vi "DB - [MasterData].[Procedure].vi"(0 "connection reference":T5, 1 "DB Connection":T1={"Open"=TRUE, "Close"=TRUE}, 2 "DB - Master Data Enum":T2, 5 "DB.Schema.Table\nSRTRS.MasterData.Procedure":string="SRTRS.MasterData.Procedure", 7 "Include Inactive":bool=TRUE, 9 "DB.Schema.Table\nSRTRS.MasterData.ProcedureItem":string="SRTRS.MasterData.ProcedureItem", 11 "error in (no error)":errorcluster, 12 "MCListbox Refnum":refnum<vi>, 13 "Clust Refnum":refnum<vi>, 14 "CmbBox Refnum":refnum<vi>) -> (4 "connection reference":T5, 6 "Result":string[](array[string]), 8 "ItemNames":string[][](array[string]), 15 "SUMMARY":errorcluster)   [LabVIEW 2013]
uses:
  <vilib>/addons/database/Connection.llb/Conn ObjectReference.ctl
  Controls/Combo Box.ctl
  Controls/DB - Master Data Procedure Enum.ctl
  Controls/DB - OpenClose.ctl
  Controls/Global SRTRS.vi
  <vilib>/addons/database/Connection.llb/DB Tools Open Connec (String).vi
  <vilib>/addons/database/Connection.llb/Conn Execute.vi
  <vilib>/addons/database/Recordset.llb/Rec Destroy - Connection.vi
  <vilib>/addons/database/Recordset.llb/Rec Fetch Recordset Data (R).vi
  <vilib>/addons/database/_DB Variant To Data/Database Variant To Data.xnode
  <vilib>/addons/database/NI_Database_API.lvlib
panel:
  out "Refnum":errorcluster
  out "Close":errorcluster
  out "Not a Refnum?":bool
  out "array w/ subset deleted":string[][](array[string])
  out "revision":string[][](array[string])
  in  "MCListBox FHS Master Data":i32(listbox)=-1 caption="Furnance Heating Sequence"
  out "SQL Statement":errorcluster
  out "ms":u32=3
  out "SQL Statement":string="USE [SRTRS]\n--GO\n\nINSERT INTO [MasterData].[Procedure]\n           ([procedureNo]\n           ,[revision]\n           ,[holdTemperture]\n           ,[unitOfMeasurement]\n           ,[holdTimeDuration]\n           ,[def]\n           ,[createdBy]\n           ,[createdOn]\n           ,[lastSavedBy]\n           ,[lastSavedOn]\n           ,[Inactive])\n     VALUES\n           ('WPS5' ,'2' ,'32' ,'°C' ,'00:02' ,'' ,'User' ,'2014-08-29 16:57:39' ,'User' ,'2014-08-29 16:57:39' ,'0' )\n--GO\n"
  in  "WPS Details Master Data":T4={"Master Data WPS/Ref"="WPS5", "Master Data Rev"="2", "Master Data Hold Temperature"="32", "Master Data Temperature Units"="°C", "Master Data Hold Time (HH:MM)"="00:02", "Inactive"=FALSE} caption="Header"
  out "procedureNo":string[][](array[string])=[["2", "1", "1", "20", "", "2014-08-29 14:24:57", "", "", "", "", "", ""]]
  out "Connection Information":T6={"Connection "="SQL Server 32bit HPEnvy", "Username"="admin", "Password"="admin123"}
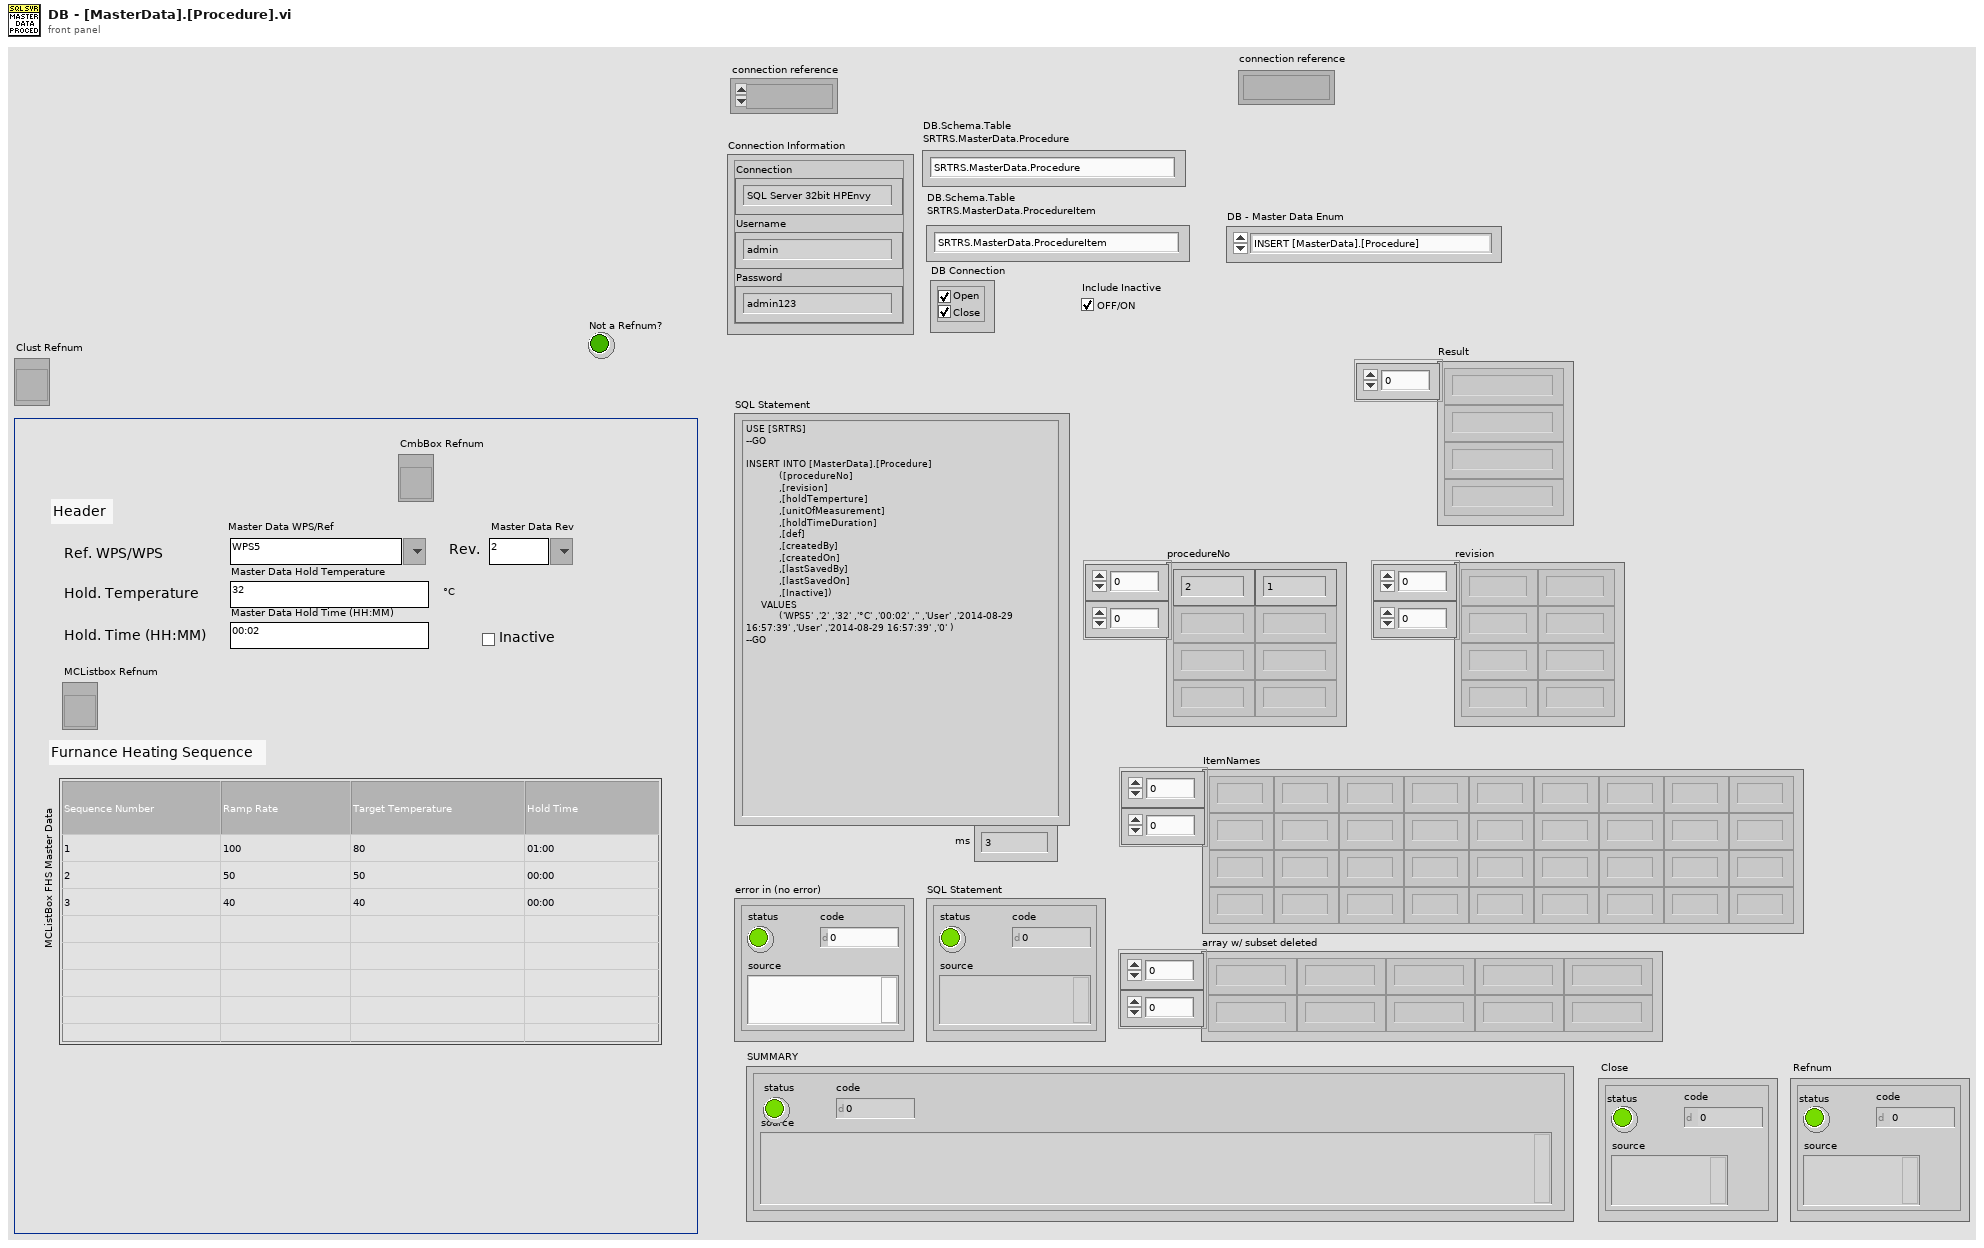
[diagram p1: front panel]
types:
  T1 = typedef "DB - OpenClose.ctl" = cluster{"Open":bool, "Close":bool}
  T2 = typedef "DB - Master Data Procedure Enum.ctl" = enum16{"INSERT [MasterData].[Procedure]", "INSERT [MasterData][ProcedureItem]", "SELECT [ProcedureNo]", "SELECT [ProcedureRev]", "SELECT [MasterData].[ProcedureItem]"}
  T3 = typedef "Combo Box.ctl" = string
  T4 = cluster{"Master Data WPS/Ref":T3, "Master Data Rev":T3, "Master Data Hold Temperature":string, "Master Data Temperature Units":string, "Master Data Hold Time (HH:MM)":string, "Inactive":bool}
  T5 = typedef "NI_Database_API.lvlib/Conn ObjectReference.ctl" = refnum<k1>
  T6 = cluster{"Connection ":string, "Username":string, "Password":string}
  T7 = typedef "Enum - InteractiveMode-SubVIMode.ctl" = enum16{"Interactive", "subVI Mode"}
  T8 = typedef "DB - Logon Info.ctl" = cluster{"PlantID":string, "SystemID":string, "UserID":string, "DomainID":string, "LanguageID":string, "StationID":string}
  T9 = typedef "Connection Information Cluster.ctl" = cluster{"Connection ":string, "Username":string, "Password":string}
  T10 = typedef "DB - DB.Schema.Table.ctl" = cluster{"DB":string, "Schema":string, "Table":string}
  T11 = typedef "NI_Database_API.lvlib/Rec ObjectReference.ctl" = refnum<k1>
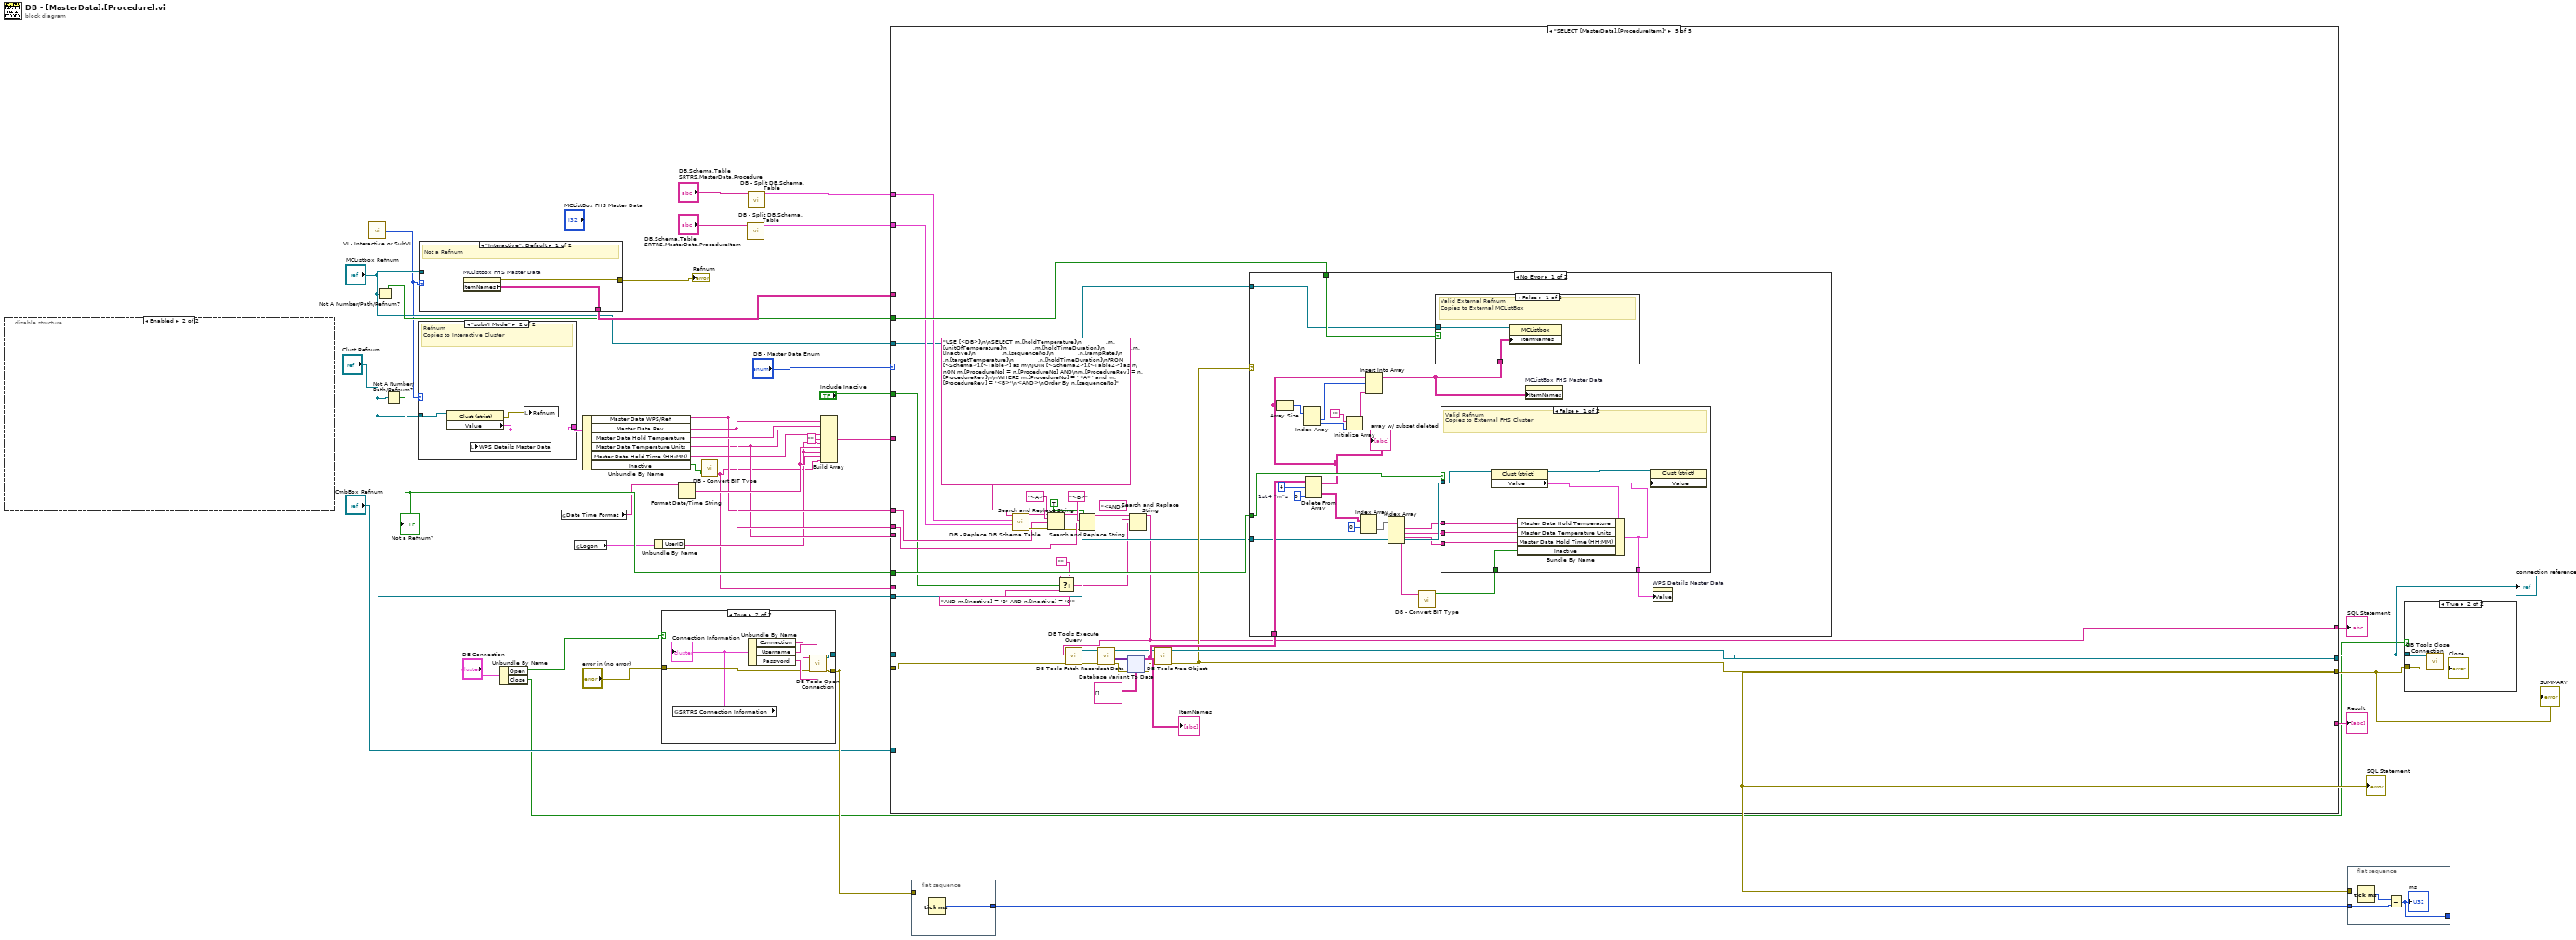
[diagram p0: block diagram]
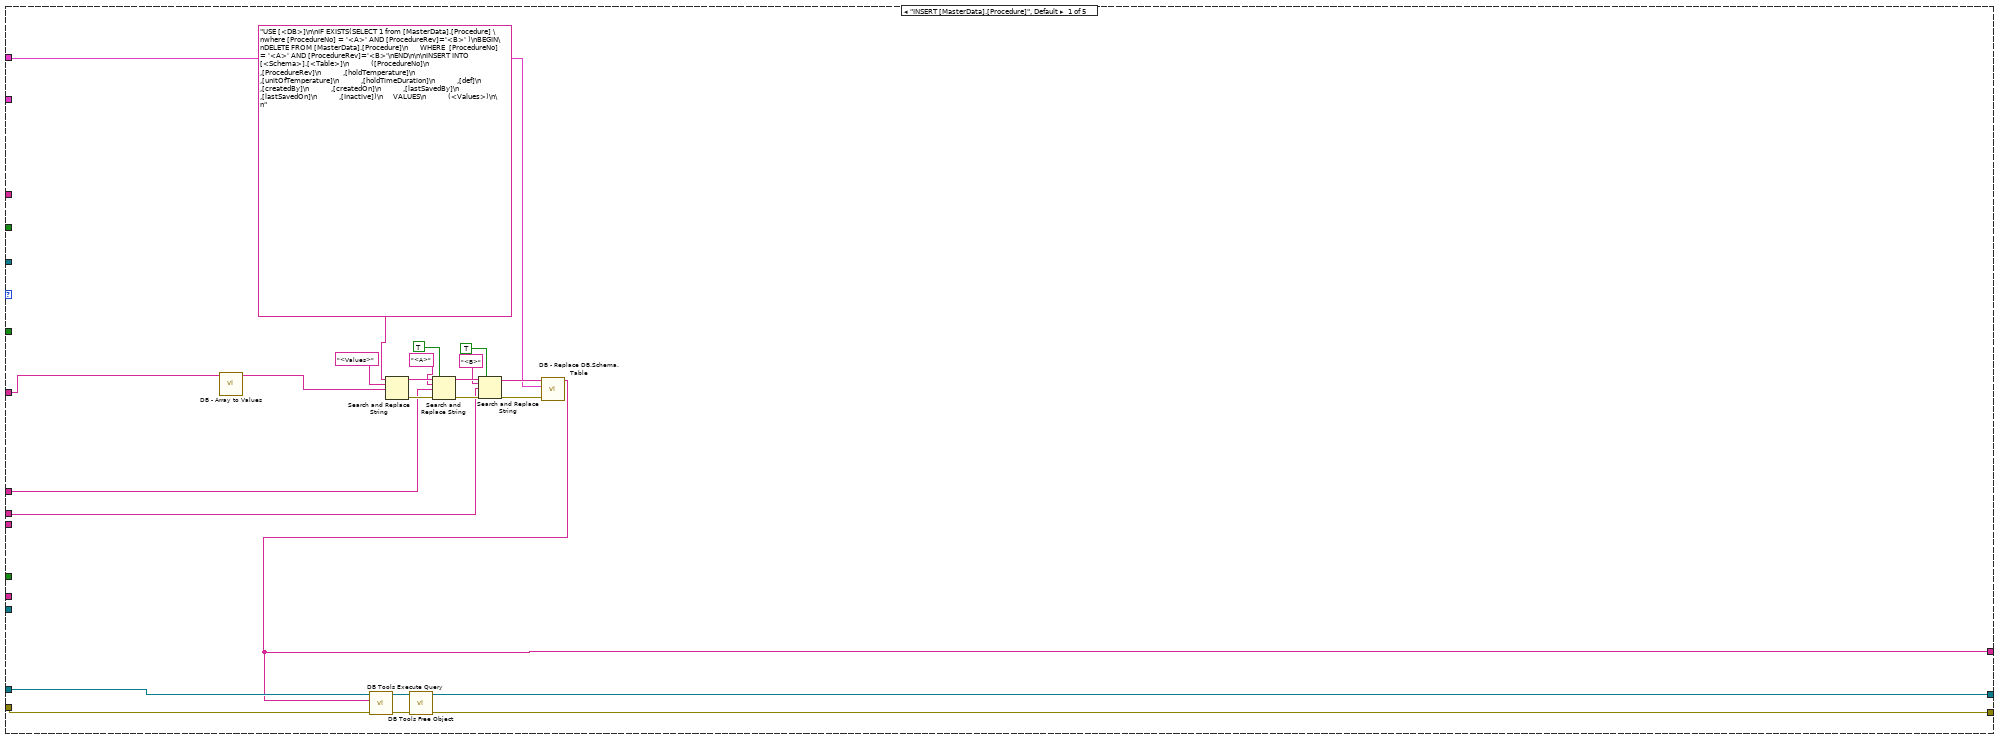
[diagram p3: hidden frame]
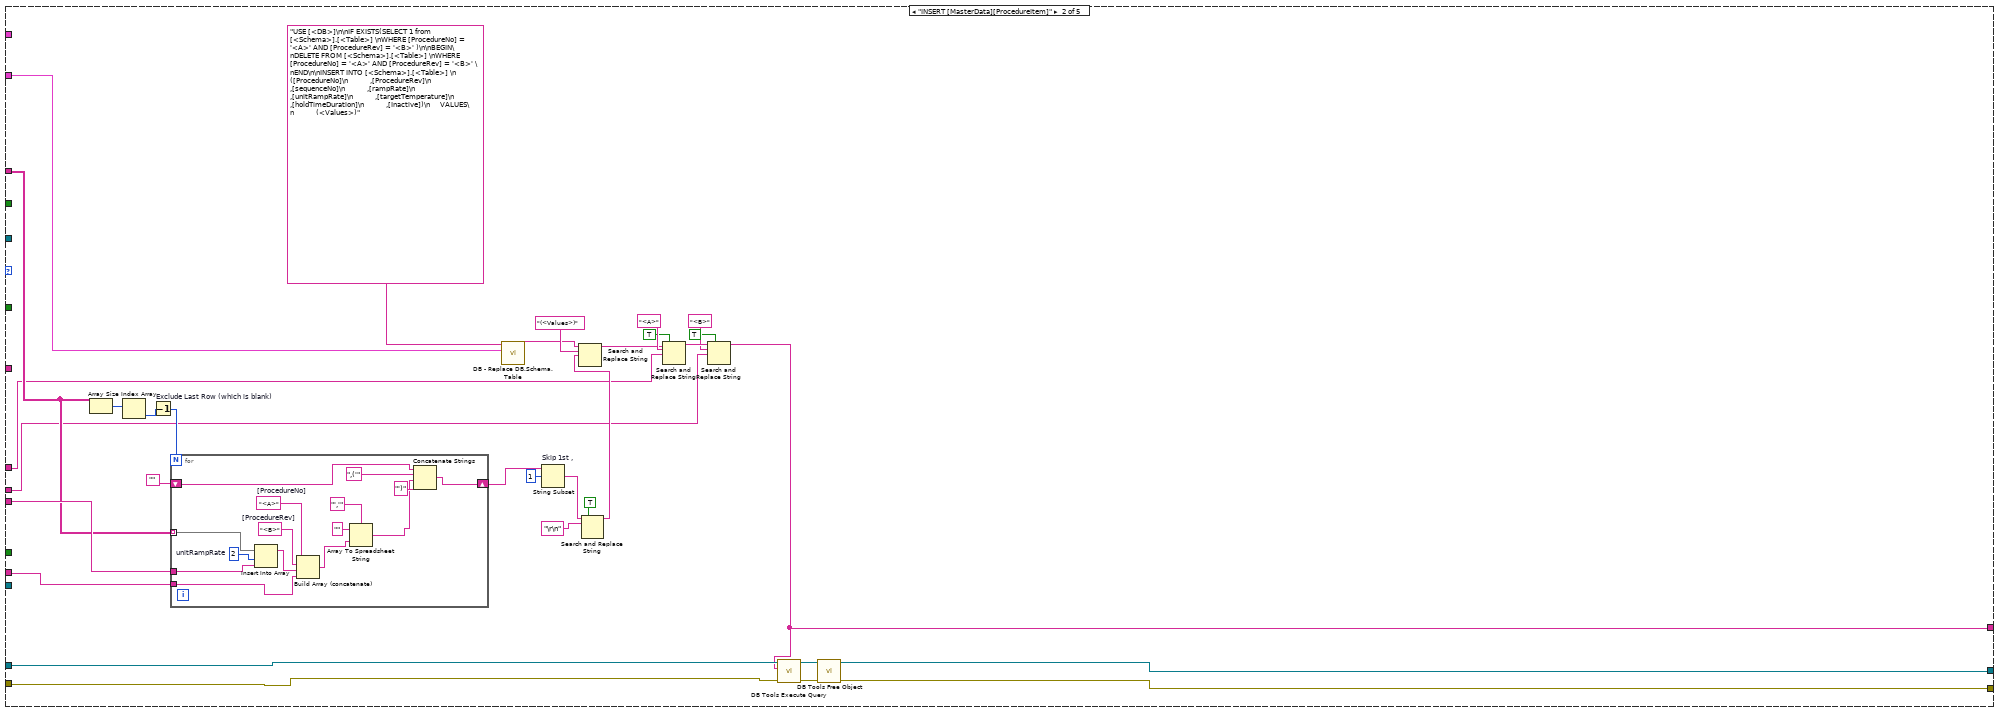
[diagram p4: hidden frame]
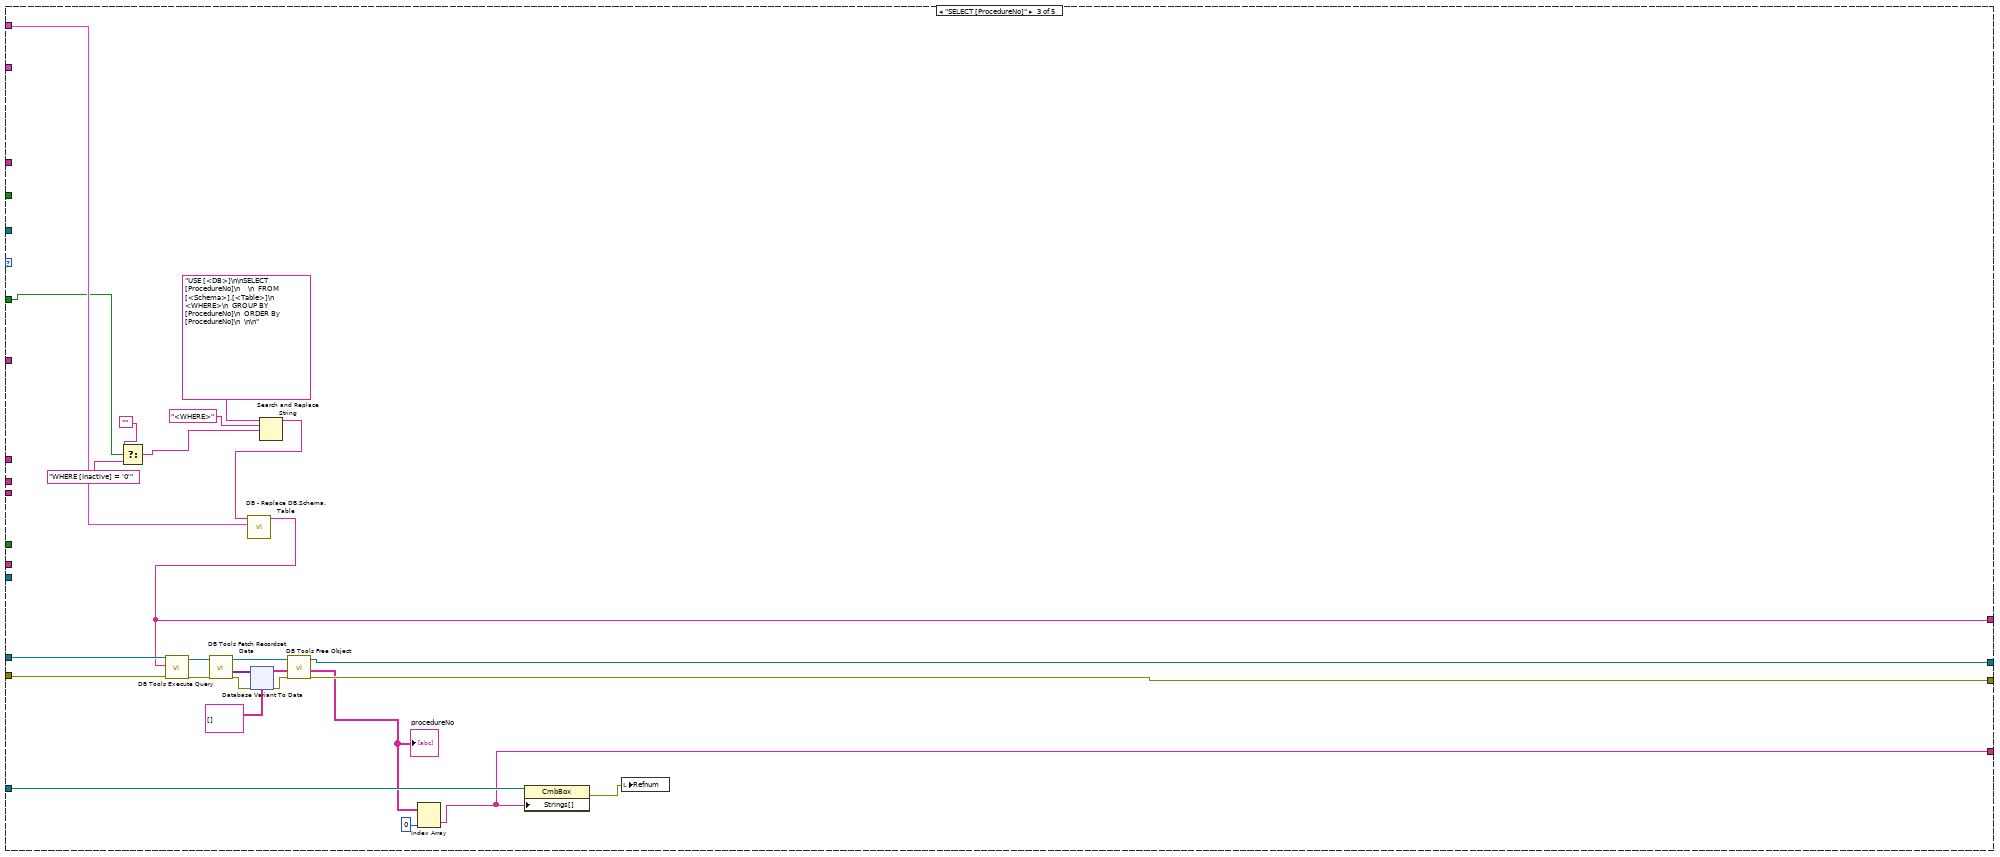
[diagram p5: hidden frame]
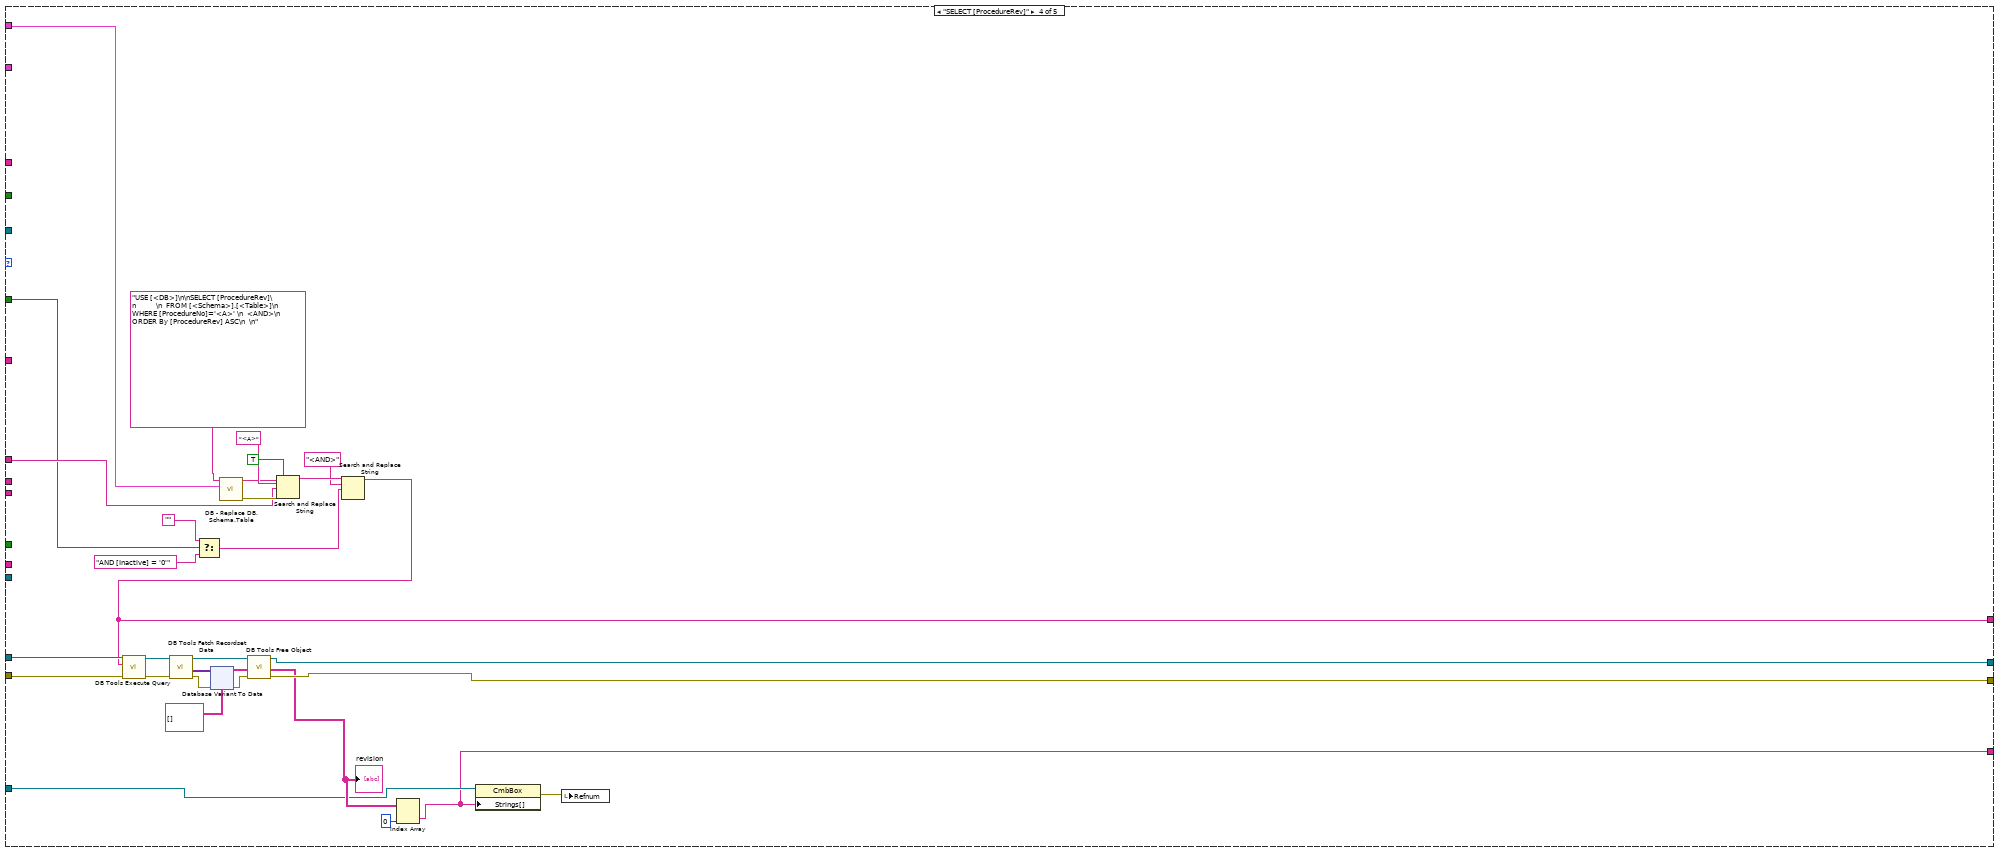
[diagram p6: hidden frame]
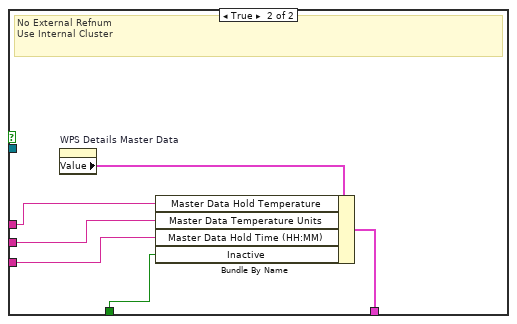
[diagram p7: hidden frame]
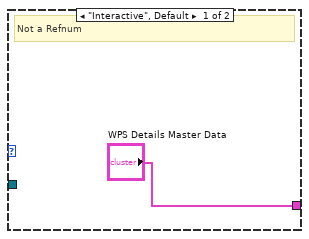
[diagram p10: hidden frame]
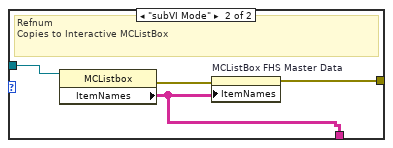
[diagram p11: hidden frame]
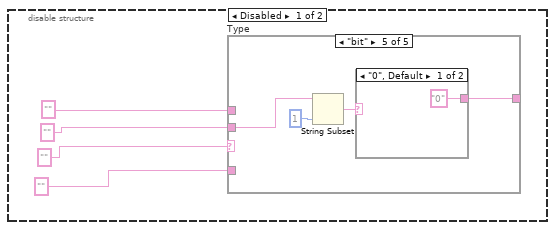
[diagram p12: hidden frame]
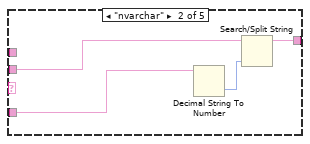
[diagram p14: hidden frame]
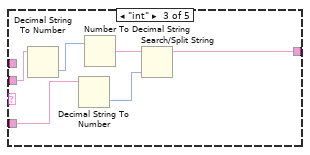
[diagram p15: hidden frame]
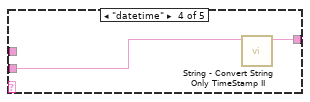
[diagram p16: hidden frame]
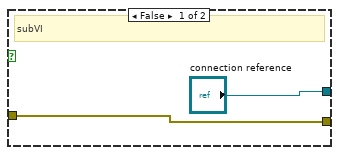
[diagram p18: hidden frame]
diagram:
  n1 = disable-structure shown="Enabled" {
    frame Disabled {
      n2 = case "Type" shown="\"bit\"" "" {
        tunnel: "" -> [w44 w47 w54 w56 w60]
        tunnel: "" -> [_ _ _ _ _]
        tunnel: "" -> [_ w46 w50 _ _]
        tunnel: [w44 w45 w49 w55 w57] -> _
        frame "False", Default {
        }
        frame "nvarchar" {
          n3 = Decimal String To Number(string=w46) -> (number=w48:i32)  [unwired: 2 in, 1 out]
          n4 = Search/Split String(string=w47, offset (0)=w48) -> (substring before match=w45:string)  [unwired: 1 in, 2 out]
        }
        frame "int" {
          n5 = Decimal String To Number(string=w54) -> (number=w53:i32)  [unwired: 2 in, 1 out]
          n6 = Decimal String To Number(string=w50) -> (number=w52:i32)  [unwired: 2 in, 1 out]
          n7 = Number To Decimal String(number=w53) -> (decimal integer string=w51:string)  [unwired: 1 in]
          n8 = Search/Split String(string=w51, offset (0)=w52) -> (substring before match=w49:string)  [unwired: 1 in, 2 out]
        }
        frame "datetime" {
          n9 = call "String - Convert String Only TimeStamp II.vi"("YYYY-mm-dd HH:MM:SS"=w56) -> ("YYYY-mm-dd HH:MM:SS"=w55:string)  [unwired: 9 in, 1 out]
        }
        frame "bit" {
          n10 = String Subset(string=w60, length (rest)=1 ("length (rest)")) -> (substring=w58:string)  [unwired: 1 in]
          n11 = case shown="\"0\", Default" w58 {
            selector: w58 -> [_ w62]
            tunnel: ["0" w62] -> w57
            frame "0", Default {
            }
            frame "1" {
            }
          }
        }
      }
    }
    frame Enabled {
    }
  }
  n12 = call "VI - Interactive or SubVI.vi"() -> ("Mode"=w9:T7)  [unwired: 5 in]
  n13 = Not A Number/Path/Refnum?(number/path/refnum="MCListbox Refnum") -> (NaN/Path/Refnum?=w19:bool)
  n14 = Not A Number/Path/Refnum?(number/path/refnum="Clust Refnum") -> (NaN/Path/Refnum?=w14:bool)
  "Not a Refnum?" <- w14
  n15 = case shown="\"subVI Mode\"" w9 {
    tunnel: "Clust Refnum" -> [_ w66]
    tunnel: ["WPS Details Master Data" w65] -> w27
    frame "Interactive", Default {
      # "Not a Refnum"
    }
    frame "subVI Mode" {
      # "Refnum\nCopies to Interactive Cluster"
      n16 = property class="Clust (strict)"(reference=w66) -> (error out=w64:errorcluster, "Value"=w65:T4)  [unwired: 1 in, 1 out]
      n17 = local write "WPS Details Master Data"(w65) -> ()
      n18 = local write "Refnum"(w64) -> ()
    }
  }
  n19 = case shown="\"Interactive\", Default" w9 {
    tunnel: "MCListbox Refnum" -> [_ w72]
    tunnel: [w68 w71] -> w22
    tunnel: [w67 w69] -> w8
    frame "Interactive", Default {
      # "Not a Refnum"
      n20 = property on="MCListBox FHS Master Data" class="MCListbox (strict)"() -> (error out=w67:errorcluster, "ItemNames"=w68:string[][])  [unwired: 2 in, 1 out]
    }
    frame "subVI Mode" {
      # "Refnum\nCopies to Interactive MCListBox"
      n21 = property class="MCListbox"(reference=w72) -> (error out=w70:errorcluster, "ItemNames"=w71:string[][])  [unwired: 1 in, 1 out]
      n22 = property on="MCListBox FHS Master Data" class="MCListbox (strict)"(error in=w70, "ItemNames"=w71) -> (error out=w69:errorcluster)  [unwired: 1 in, 1 out]
    }
  }
  "Refnum" <- w8
  n23 = Unbundle By Name("DB Connection") -> ("Open"=w3:bool, "Close"=w2:bool)
  n24 = global read "Global SRTRS.vi" "Date Time Format"() -> (w7:string)
  n25 = global read "Global SRTRS.vi" "Logon"() -> (w6:T8)
  n26 = Unbundle By Name(w27) -> ("Master Data WPS/Ref"=w24:T3, "Master Data Rev"=w25:T3, "Master Data Hold Temperature"=w36:string, "Master Data Temperature Units"=w21:string, "Master Data Hold Time (HH:MM)"=w35:string, "Inactive"=w12:bool)
  n27 = Unbundle By Name(w6) -> ("UserID"=w5:string)
  n28 = case shown="True" w3 {
    tunnel: ["connection reference" w78] -> w37
    tunnel: "error in (no error)" -> [w73 w77]
    tunnel: [w73 w76] -> w28
    frame False {
      # "subVI"
    }
    frame True {
      n29 = global read "Global SRTRS.vi" "SRTRS Connection Information"() -> (w75:T9)
      "Connection Information" <- w75
      n30 = Unbundle By Name(w75) -> ("Connection"=w80:string, "Username"=w81:string, "Password"=w79:string)
      n31 = call-poly <vilib>:"DB Tools Open Connection.vi"("password"=w79, "userID"=w81, "error in (no error)"=w77, "connection information"=w80) -> ("error out"=w76:errorcluster, "connection reference"=w78:T5)  [unwired: 4 in]
    }
  }
  n32 = Format Date/Time String(time format string (%c)=w7) -> (date/time string=w31:string)  [unwired: 2 in]
  n33 = call "DB - Convert BIT Type.vi"("Boolean"=w12) -> ("BIT (eg Inactive)"=w1:string)  [unwired: 2 in, 2 out]
  n34 = call "DB - Split DB.Schema.Table.vi"("DB.Schema.Table"="DB.Schema.Table\nSRTRS.MasterData.ProcedureItem") -> ("DB.Schema.Table"=w18:T10)  [unwired: 10 in]
  n35 = call "DB - Split DB.Schema.Table.vi"("DB.Schema.Table"="DB.Schema.Table\nSRTRS.MasterData.Procedure") -> ("DB.Schema.Table"=w26:T10)  [unwired: 10 in]
  n36 = Build Array(w24, w25, w36, w21, w35, "" ("string"), w5, w31, w5, w31, w1) -> (w33:T3[])
  n37 = case shown="\"SELECT [MasterData].[ProcedureItem]\"" "DB - Master Data Enum" {
    tunnel: [w105 w124 w168 w237 w314] -> w20
    tunnel: w37 -> [w104 w113 w170 w239 w316]
    tunnel: w33 -> [w102 _ _ _ _]
    tunnel: [w100 w107 w166 w228 w297] -> w32
    tunnel: w28 -> [w99 w115 w169 w238 w315]
    tunnel: w26 -> [w87 _ w165 w234 w311]
    tunnel: [w86 w123 w167 w236 w312] -> w10
    tunnel: w25 -> [w85 w116 _ _ w308]
    tunnel: w24 -> [w84 w117 _ w235 w309]
    tunnel: w22 -> [_ w121 _ _ _]
    tunnel: w21 -> [_ w122 _ _ _]
    tunnel: w19 -> [_ _ _ _ w313]
    tunnel: w18 -> [_ w110 _ _ w310]
    tunnel: "MCListbox Refnum" -> [_ _ _ _ w307]
    tunnel: "CmbBox Refnum" -> [_ _ w164 w231 _]
    tunnel: [_ _ w161 w230 _] -> w15
    tunnel: w14 -> [_ _ _ _ w304]
    tunnel: "Clust Refnum" -> [_ _ _ _ w303]
    tunnel: "Include Inactive" -> [_ _ w156 w225 w300]
    tunnel: w1 -> [_ w106 _ _ _]
    frame "INSERT [MasterData].[Procedure]", Default {
      n38 = call "DB - Array to Values.vi"("Array (0xFFFE autodetect)"=w102) -> ("<Values>"=w101:string)  [unwired: 10 in]
      n39 = Search and Replace String(input string="USE [<DB>]\n\nIF EXISTS(SELECT 1 from [MasterData].[Procedure] \nwhere [ProcedureNo] = '<A>' AND [ProcedureRev]='<B>' )\nBEGIN\nDELETE FROM [MasterData].[Procedure]\n      WHERE  [ProcedureNo] = '<A>' AND [ProcedureRev]='<B>'\nEND\n\n\nINSERT INTO [<Schema>].[<Table>]\n           ([ProcedureNo]\n           ,[ProcedureRev]\n           ,[holdTemperature]\n           ,[unitOfTemperature]\n           ,[holdTimeDuration]\n           ,[def]\n           ,[createdBy]\n           ,[createdOn]\n           ,[lastSavedBy]\n           ,[lastSavedOn]\n           ,[Inactive])\n     VALUES\n           (<Values>)\n\n", search string="<Values>", replace string=w101) -> (result string=w94:string, error out=w97:errorcluster)  [unwired: 5 in, 2 out]
      n40 = Search and Replace String(replace all?=TRUE ("replace all? (F)"), input string=w94, search string="<A>" ("input string"), replace string=w84, error in=w97) -> (result string=w93:string, error out=w96:errorcluster)  [unwired: 3 in, 2 out]
      n41 = Search and Replace String(replace all?=TRUE ("replace all? (F)"), input string=w93, search string="<B>" ("input string"), replace string=w85, error in=w96) -> (result string=w90:string, error out=w95:errorcluster)  [unwired: 3 in, 2 out]
      n42 = call "DB - Replace DB.Schema.Table.vi"("error in (no error)"=w95, "DB.Schema.Table"=w87, "string in"=w90) -> ("string out"=w100:string)  [unwired: 7 in, 1 out]
      n43 = call-poly <vilib>:"DB Tools Execute Query.vi"("error in (no error)"=w99, "SQL query"=w100, "connection reference"=w104) -> ("error out"=w82:errorcluster, "recordset reference"=w83:T11)  [unwired: 5 in]
      n44 = call-poly <vilib>:"DB Tools Free Object.vi"("error in (no error)"=w82, "recordset reference"=w83) -> ("error out"=w86:errorcluster, "connection reference"=w105:T5)  [unwired: 8 in]
    }
    frame "INSERT [MasterData][ProcedureItem]" {
      n45 = Array Size(array=w121) -> (size(s)=w131:i32[])
      n46 = Index Array(array=w131) -> (element=w132:i32)  [unwired: 1 in]
      n47 = Decrement "Exclude Last Row (which is blank)"(x=w132) -> (x-1=w133:i32)
      n48 = for {
        N: w133 -> [_]
        tunnel: w121 -> [w144] mode=indexing
        shift-right: [w147] -> w126
        shift-left: "" -> [w148]
        tunnel: w122 -> [w143]
        tunnel: w106 -> [w138]
        w139 = "<B>"  # [ProcedureRev]
        w140 = "<A>"  # [ProcedureNo]
        w145 = 2  # unitRampRate
        n49 = Insert Into Array(array=w144, index=w145, new element=w143) -> (w142:string[])
        n50 = Build Array (concatenate)(w140, w139, w142, w138) -> (w141:string[])
        n51 = Array To Spreadsheet String(delimiter (Tab)="','", array=w141, 3:"" ("format string")) -> (spreadsheet string=w146:string)
        n52 = Concatenate Strings(w148, ",('" ("string"), w146, "')" ("string")) -> (w147:string)
      }
      n53 = call "DB - Replace DB.Schema.Table.vi"("DB.Schema.Table"=w110, "string in"="USE [<DB>]\n\nIF EXISTS(SELECT 1 from [<Schema>].[<Table>] \nWHERE [ProcedureNo] = '<A>' AND [ProcedureRev] = '<B>' )\n\nBEGIN\nDELETE FROM [<Schema>].[<Table>] \nWHERE [ProcedureNo] = '<A>' AND [ProcedureRev] = '<B>' \nEND\n\nINSERT INTO [<Schema>].[<Table>] \n           ([ProcedureNo]\n           ,[ProcedureRev]\n           ,[sequenceNo]\n           ,[rampRate]\n           ,[unitRampRate]\n           ,[targetTemperature]\n           ,[holdTimeDuration]\n           ,[Inactive])\n     VALUES\n           (<Values>)") -> ("string out"=w109:string)  [unwired: 8 in, 1 out]
      n54 = String Subset "Skip 1st ,"(string=w126, offset (0)=1) -> (substring=w128:string)  [unwired: 1 in]
      n55 = Search and Replace String(replace all?=TRUE ("replace all? (F)"), input string=w128, search string="\r\n") -> (result string=w135:string)  [unwired: 5 in, 3 out]
      n56 = Search and Replace String(input string=w109, search string="(<Values>)", replace string=w135) -> (result string=w108:string)  [unwired: 5 in, 3 out]
      n57 = Search and Replace String(replace all?=TRUE ("replace all? (F)"), input string=w108, search string="<A>", replace string=w117) -> (result string=w120:string)  [unwired: 4 in, 3 out]
      n58 = Search and Replace String(replace all?=TRUE ("replace all? (F)"), input string=w120, search string="<B>", replace string=w116) -> (result string=w107:string)  [unwired: 4 in, 3 out]
      n59 = call-poly <vilib>:"DB Tools Execute Query.vi"("error in (no error)"=w115, "SQL query"=w107, "connection reference"=w113) -> ("error out"=w137:errorcluster, "recordset reference"=w136:T11)  [unwired: 5 in]
      n60 = call-poly <vilib>:"DB Tools Free Object.vi"("error in (no error)"=w137, "recordset reference"=w136) -> ("error out"=w123:errorcluster, "connection reference"=w124:T5)  [unwired: 8 in]
    }
    frame "SELECT [ProcedureNo]" {
      n61 = Select(t="", s=w156, f="WHERE [Inactive] = '0'" ("search string")) -> (s? t:f=w154:string)
      n62 = Search and Replace String(input string="USE [<DB>]\n\nSELECT [ProcedureNo]\n    \n  FROM [<Schema>].[<Table>]\n  <WHERE>\n  GROUP BY [ProcedureNo]\n  ORDER By [ProcedureNo]\n  \n\n", search string="<WHERE>", replace string=w154) -> (result string=w158:string)  [unwired: 5 in, 3 out]
      n63 = call "DB - Replace DB.Schema.Table.vi"("DB.Schema.Table"=w165, "string in"=w158) -> ("string out"=w166:string)  [unwired: 8 in, 1 out]
      n64 = call-poly <vilib>:"DB Tools Execute Query.vi"("error in (no error)"=w169, "SQL query"=w166, "connection reference"=w170) -> ("error out"=w173:errorcluster, "recordset reference"=w177:T11)  [unwired: 5 in]
      n65 = call-poly <vilib>:"DB Tools Fetch Recordset Data.vi"("error in (no error)"=w173, "recordset reference"=w177) -> ("error out"=w176:errorcluster, "recordset data"=w172:variant[][], "recordset reference out"=w174:T11)  [unwired: 3 in]
      n66 = xnode "Database Variant To Data"("database variant"=w172, "error in (no error)"=w176, "type"=string[][] []) -> ("data"=w163:string[][], "error out"=w171:errorcluster)
      "procedureNo" <- w163
      n67 = call-poly <vilib>:"DB Tools Free Object.vi"("error in (no error)"=w171, "recordset reference"=w174) -> ("error out"=w167:errorcluster, "connection reference"=w168:T5)  [unwired: 8 in]
      n68 = Index Array(array=w163, index (col)=0 ("disabled index (col)")) -> (element=w161:string[])  [unwired: 1 in]
      n69 = property class="CmbBox"(reference=w164, "Strings[]"=w161) -> (error out=w153:errorcluster)  [unwired: 1 in, 1 out]
      n70 = local write "Refnum"(w153) -> ()
    }
    frame "SELECT [ProcedureRev]" {
      n71 = Select(t="", s=w225, f="AND [Inactive] = '0'") -> (s? t:f=w223:string)
      n72 = call "DB - Replace DB.Schema.Table.vi"("DB.Schema.Table"=w234, "string in"="USE [<DB>]\n\nSELECT [ProcedureRev]\n          \n  FROM [<Schema>].[<Table>]\n  WHERE [ProcedureNo]='<A>' \n  <AND>\n  ORDER By [ProcedureRev] ASC\n  \n") -> ("error out"=w244:errorcluster, "string out"=w241:string)  [unwired: 8 in]
      n73 = Search and Replace String(replace all?=TRUE ("replace all? (F)"), input string=w241, search string="<A>", replace string=w235, error in=w244) -> (result string=w229:string)  [unwired: 3 in, 3 out]
      n74 = Search and Replace String(input string=w229, search string="<AND>", replace string=w223) -> (result string=w228:string)  [unwired: 5 in, 3 out]
      n75 = call-poly <vilib>:"DB Tools Execute Query.vi"("error in (no error)"=w238, "SQL query"=w228, "connection reference"=w239) -> ("error out"=w249:errorcluster, "recordset reference"=w245:T11)  [unwired: 5 in]
      n76 = call-poly <vilib>:"DB Tools Fetch Recordset Data.vi"("error in (no error)"=w249, "recordset reference"=w245) -> ("error out"=w246:errorcluster, "recordset data"=w250:variant[][], "recordset reference out"=w248:T11)  [unwired: 3 in]
      n77 = xnode "Database Variant To Data"("database variant"=w250, "error in (no error)"=w246, "type"=string[][] []) -> ("data"=w233:string[][], "error out"=w251:errorcluster)
      "revision" <- w233
      n78 = call-poly <vilib>:"DB Tools Free Object.vi"("error in (no error)"=w251, "recordset reference"=w248) -> ("error out"=w236:errorcluster, "connection reference"=w237:T5)  [unwired: 8 in]
      n79 = Index Array(array=w233, index (col)=0 ("disabled index (col)")) -> (element=w230:string[])  [unwired: 1 in]
      n80 = property class="CmbBox"(reference=w231, "Strings[]"=w230) -> (error out=w222:errorcluster)  [unwired: 1 in, 1 out]
      n81 = local write "Refnum"(w222) -> ()
    }
    frame "SELECT [MasterData].[ProcedureItem]" {
      w305 = TRUE ("replace all? (F)")
      n82 = call "DB - Replace DB.Schema.Table.vi"("DB.Schema.Table 2"=w310, "DB.Schema.Table"=w311, "string in"="USE [<DB>]\n\nSELECT m.[holdTemperature]\n             ,m.[unitOfTemperature]\n              ,m.[holdTimeDuration]\n              ,m.[Inactive]\n              ,n.[sequenceNo]\n             ,n.[rampRate]\n             ,n.[targetTemperature]\n             ,n.[holdTimeDuration]\nFROM [<Schema>].[<Table>] as m\nJOIN [<Schema2>].[<Table2>] as n\nON m.[ProcedureNo] = n.[ProcedureNo] AND\nm.[ProcedureRev] = n.[ProcedureRev]\n\nWHERE m.[ProcedureNo] = '<A>' and m.[ProcedureRev] = '<B>'\n<AND>\nOrder By n.[sequenceNo]") -> ("error out"=w327:errorcluster, "string out"=w325:string)  [unwired: 7 in]
      n83 = Search and Replace String(replace all?=w305, input string=w325, search string="<A>", replace string=w309, error in=w327) -> (result string=w328:string, error out=w306:errorcluster)  [unwired: 3 in, 2 out]
      n84 = Select(t="", s=w300, f="AND m.[Inactive] = '0' AND n.[Inactive] = '0'" ("search string")) -> (s? t:f=w299:string)
      n85 = Search and Replace String(replace all?=w305, input string=w328, search string="<B>", replace string=w308, error in=w306) -> (result string=w298:string)  [unwired: 3 in, 3 out]
      n86 = Search and Replace String(input string=w298, search string="<AND>", replace string=w299) -> (result string=w297:string)  [unwired: 5 in, 3 out]
      n87 = call-poly <vilib>:"DB Tools Execute Query.vi"("error in (no error)"=w315, "SQL query"=w297, "connection reference"=w316) -> ("error out"=w319:errorcluster, "recordset reference"=w323:T11)  [unwired: 5 in]
      n88 = call-poly <vilib>:"DB Tools Fetch Recordset Data.vi"("error in (no error)"=w319, "recordset reference"=w323) -> ("error out"=w322:errorcluster, "recordset data"=w318:variant[][], "recordset reference out"=w320:T11)  [unwired: 3 in]
      n89 = xnode "Database Variant To Data"("database variant"=w318, "error in (no error)"=w322, "type"=string[][] []) -> ("data"=w330:string[][], "error out"=w317:errorcluster)
      "ItemNames" <- w330
      n90 = call-poly <vilib>:"DB Tools Free Object.vi"("error in (no error)"=w317, "recordset reference"=w320) -> ("error out"=w312:errorcluster, "connection reference"=w314:T5)  [unwired: 8 in]
      n91 = case shown="No Error" w312 {
        tunnel: w330 -> [w345 _]
        tunnel: w313 -> [w353 _]
        tunnel: w307 -> [w346 _]
        tunnel: w304 -> [w342 _]
        tunnel: w303 -> [w341 _]
        frame No Error {
          w343 = 4  # 1st 4 "m"s
          n92 = Delete From Array(array=w345, length=w343, index (col)=0 ("disabled index (col)")) -> (deleted portion=w333:string[][], array with subset deleted=w338:string[][])  [unwired: 1 in]
          "array w/ subset deleted" <- w338
          n93 = Array Size(array=w338) -> (size(s)=w352:i32[])
          n94 = Index Array(array=w352) -> (element #1=w349:i32, element #2=w351:i32)  [unwired: 2 in]
          n95 = Initialize Array("", w351) -> (w348:string[])
          n96 = Index Array(array=w333, index (row)=0) -> (element=w340:string[])  [unwired: 1 in]
          n97 = Insert Into Array(array=w338, index (row)=w349, new element=w348) -> (w347:string[][])  [unwired: 1 in]
          n98 = Index Array(array=w340) -> (element #1=w337:string, element #2=w336:string, element #3=w335:string, element #4=w332:string)  [unwired: 4 in]
          n99 = call "DB - Convert BIT Type.vi"("BIT Type (eg Inactive)"=w332) -> ("Boolean"=w331:bool)  [unwired: 2 in, 2 out]
          n100 = case shown="False" w353 {
            tunnel: w347 -> [w369 _]
            tunnel: w346 -> [w368 _]
            frame False {
              # "Valid External Refnum\nCopies to External MCListBox"
              n101 = property class="MCListbox"(reference=w368, "ItemNames"=w369) -> ()  [unwired: 1 in, 2 out]
            }
            frame True {
              # "No External Refnum"
            }
          }
          n102 = case shown="False" w342 {
            tunnel: w341 -> [w361 _]
            tunnel: w337 -> [w359 w366]
            tunnel: w336 -> [w358 w365]
            tunnel: w335 -> [w357 w364]
            tunnel: [w356 w363] -> w334
            tunnel: w331 -> [w355 w362]
            frame False {
              # "Valid Refnum\nCopies to External FHS Cluster"
              n103 = property class="Clust (strict)"(reference=w361) -> (reference out=w360:refnum<vi>, "Value"=w354:T4)  [unwired: 1 in, 1 out]
              n104 = Bundle By Name(cluster=w354, "Master Data Hold Temperature"=w359, "Master Data Temperature Units"=w358, "Master Data Hold Time (HH:MM)"=w357, "Inactive"=w355) -> (w356:T4)
              n105 = property class="Clust (strict)"(reference=w360, "Value"=w356) -> ()  [unwired: 1 in, 2 out]
            }
            frame True {
              # "No External Refnum\nUse Internal Cluster"
              n106 = property on="WPS Details Master Data" class="Clust (strict)"() -> ("Value"=w367:T4)  [unwired: 2 in, 2 out]
              n107 = Bundle By Name(cluster=w367, "Master Data Hold Temperature"=w366, "Master Data Temperature Units"=w365, "Master Data Hold Time (HH:MM)"=w364, "Inactive"=w362) -> (w363:T4)
            }
          }
          n108 = property on="MCListBox FHS Master Data" class="MCListbox (strict)"("ItemNames"=w347) -> ()  [unwired: 2 in, 2 out]
          n109 = property on="WPS Details Master Data" class="Clust (strict)"("Value"=w334) -> ()  [unwired: 2 in, 2 out]
        }
        frame Error {
        }
      }
    }
  }
  "SQL Statement" <- w10
  "SQL Statement" <- w32
  "SUMMARY" <- w10
  "connection reference" <- w20
  "Result" <- w15
  n110 = flat-sequence {
    tunnel: [w414] -> w29
    tunnel: w28 -> [_]
    frame #0 {
      n111 = Tick Count (ms)() -> (millisecond timer value=w414:u32)
    }
  }
  n112 = flat-sequence {
    tunnel: w29 -> [w417]
    tunnel: [w416] -> _
    tunnel: w10 -> [_]
    frame #0 {
      n113 = Tick Count (ms)() -> (millisecond timer value=w415:u32)
      n114 = Subtract(x=w415, y=w417) -> (x-y=w416:u32)
      "ms" <- w416
    }
  }
  n115 = case shown="True" w2 {
    tunnel: w20 -> [_ w420]
    tunnel: w10 -> [_ w419]
    frame False {
      # "subVI"
    }
    frame True {
      n116 = call <vilib>:"DB Tools Close Connection.vi"("error in (no error)"=w419, "connection reference"=w420) -> ("error out"=→"Close":errorcluster)  [unwired: 5 in]
    }
  }
